vi "TimeStringToNumber.vi"(11 "time":string) -> (3 "sec":i32)   [LabVIEW 2018]
panel:
  out "min:seg":string
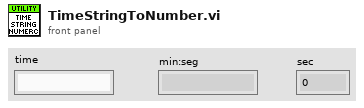
[diagram p1: front panel]
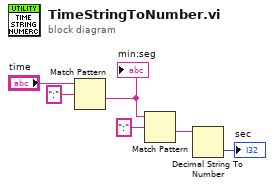
[diagram p0: block diagram]
diagram:
  n1 = Match Pattern(string="time", regular expression=":") -> (after substring=w2:string)  [unwired: 1 in, 3 out]
  "min:seg" <- w2
  n2 = Match Pattern(string=w2, regular expression=":") -> (after substring=w1:string)  [unwired: 1 in, 3 out]
  n3 = Decimal String To Number(string=w1) -> (number=→"sec":i32)  [unwired: 2 in, 1 out]
